vi "Decode MUX Values.vi"(8 "error in (no error)":errorcluster, 10 "MUX Value":i32, 11 "VISA resource name":refnum<visa-resource-name>) -> (0 "error out":errorcluster, 2 "Channels":i32[](array[ring]) items=["Channel A"=1, "Channel B"=2, "Channel C"=3, "Channel D"=4, "Channel E"=5, "Channel F"=6, "Channel G"=7, "Channel H"=8], 3 "VISA resource name out":refnum<visa-resource-name>)   [LabVIEW 2012, in "Quantum Composers 9000 Series.lvlib"]
doc: "This utility VI can be used to decode a MUX value to the individually multiplexed channels."
uses:
  <instrlib>/Quantum Composers 9000 Series/Quantum Composers 9000 Series.lvlib
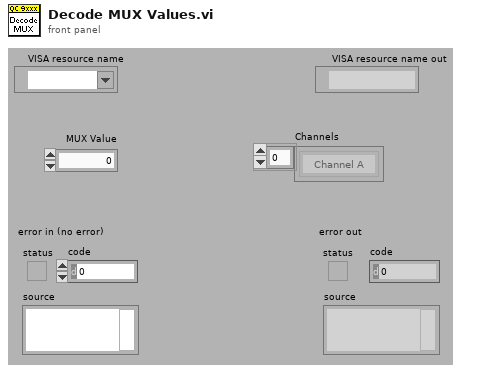
[diagram p1: front panel]
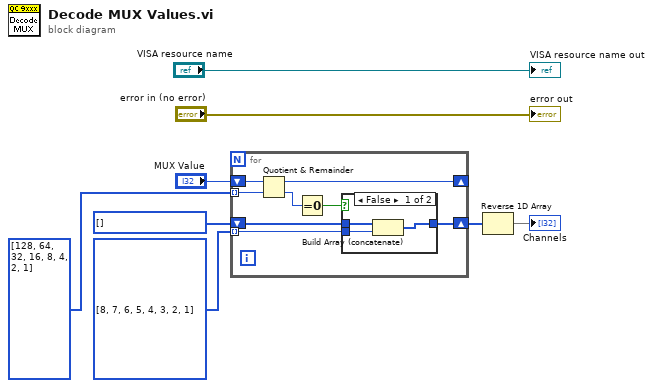
[diagram p0: block diagram]
diagram:
  w6 = i32[] [] items=["Channel A"=1, "Channel B"=2, "Channel C"=3, "Channel D"=4, "Channel E"=5, "Channel F"=6, "Channel G"=7, "Channel H"=8] ("MUX Chanels In")
  w5 = i32[] [8, 7, 6, 5, 4, 3, 2, 1] items=["Channel A"=1, "Channel B"=2, "Channel C"=3, "Channel D"=4, "Channel E"=5, "Channel F"=6, "Channel G"=7, "Channel H"=8] ("MUX Chanels In")
  n1 = for {
    shift-right: [w12] -> _
    shift-left: "MUX Value" -> [w16]
    tunnel: i32[] [128, 64, 32, 16, 8, 4, 2, 1] ("Array") -> [w15] mode=indexing
    shift-right: [w10] -> w4
    shift-left: w6 -> [w11]
    tunnel: w5 -> [w9] mode=indexing
    n2 = Quotient & Remainder(x=w16, y=w15) -> (x-y*floor(x/y)=w12:i32, floor(x/y)=w14:i32)
    n3 = Equal To 0?(x=w14) -> (x = 0?=w13:bool)
    n4 = case shown="False" w13 {
      tunnel: w11 -> [w19 w20]
      tunnel: [w18 w20] -> w10
      tunnel: w9 -> [w17 _]
      frame False {
        n5 = Build Array (concatenate)(w19, w17) -> (w18:i32[])
      }
      frame True {
      }
    }
  }
  n6 = Reverse 1D Array(array=w4) -> (reversed array=→"Channels":i32[])
  "VISA resource name out" <- "VISA resource name"
  "error out" <- "error in (no error)"
